vi "Autonomous.vi"   [LabVIEW 2018]
doc: "This VI starts when autonomous period begins, and will automatically be terminated when it ends. You can carry out timed or sensor driven operations directly to I/O or to subsystems without needing to return to the caller."
uses:
  <vilib>/Rock Robotics/WPI/DriverStation/WPI_DriverStationDerivedRobotMode.ctl
  <vilib>/Rock Robotics/Network Tables/NT Read String.vi
  Auton/Auton Kill Switch.vi
types:
  T1 = typedef "ADIS16470 Device Reference.ctl" = cluster{"DevStatus":errorcluster, "Hardware Config":T2, "End Calibration":refnum<notifier>, "Calibration Complete":refnum<notifier>, "Data FIFO":refnum<k33>, "Status FIFO":refnum<k33>, "Last Value Reference":refnum<data-value>, "Sychronous Process VI":T6, "Cmd FIFO":refnum<k33>}
  T2 = typedef "ADIS16470 Hardware Configuration.ctl" = cluster{"SPI Clock Rate (Hz)":dbl, "IMU SPI Mode (3)":T3, "IMU Reset Pin":T4, "IMU SPI Bus":T5, "IMU Data Ready Pin":T4}
  T3 = typedef "WPI_SPIMode.ctl" = enum16{"Mode 0 (Clk Idle Low,Sample on Leading)", "Mode 1 (Clk Idle Low,Sample on Trailing)", "Mode 2 (Clk Idle High,Sample on Leading)", "Mode 3 (Clk Idle High,Sample on Trailing)"}
  T4 = typedef "FPGA_DIOChannel.ctl" = enum8{"DIO 0", "DIO 1", "DIO 2", "DIO 3", "DIO 4", "DIO 5", "DIO 6", "DIO 7", "DIO 8", "DIO 9", "DIO MXP 0", "DIO MXP 1", "DIO MXP 2", "DIO MXP 3", "DIO MXP 4", "DIO MXP 5", "DIO MXP 6", "DIO MXP 7", "DIO MXP 8", "DIO MXP 9", "DIO MXP 10", "DIO MXP 11", "DIO MXP 12", "DIO MXP 13", "DIO MXP 14", "DIO MXP 15", "SPI Port CS1", "SPI Port CS2", "SPI Port CS3", "SPI Port MISO", "SPI Port MOSI", "Invalid"}
  T5 = typedef "spi_bus.ctl" = enum16{"SPI On-Board, CS0", "SPI On-Board, CS1", "SPI On-Board, CS2", "SPI On-Board, CS3", "SPI MXP", "Invalid"}
  T6 = typedef "ADIS16470 Process.ctl" = refnum<vi>
  T7 = typedef "ADIS16470 Status.ctl" = cluster{"Calibrated?":bool}
  T8 = typedef "WPI_DriverStationDerivedRobotMode.ctl" = enum16{"Init", "Execute", "Stop"}
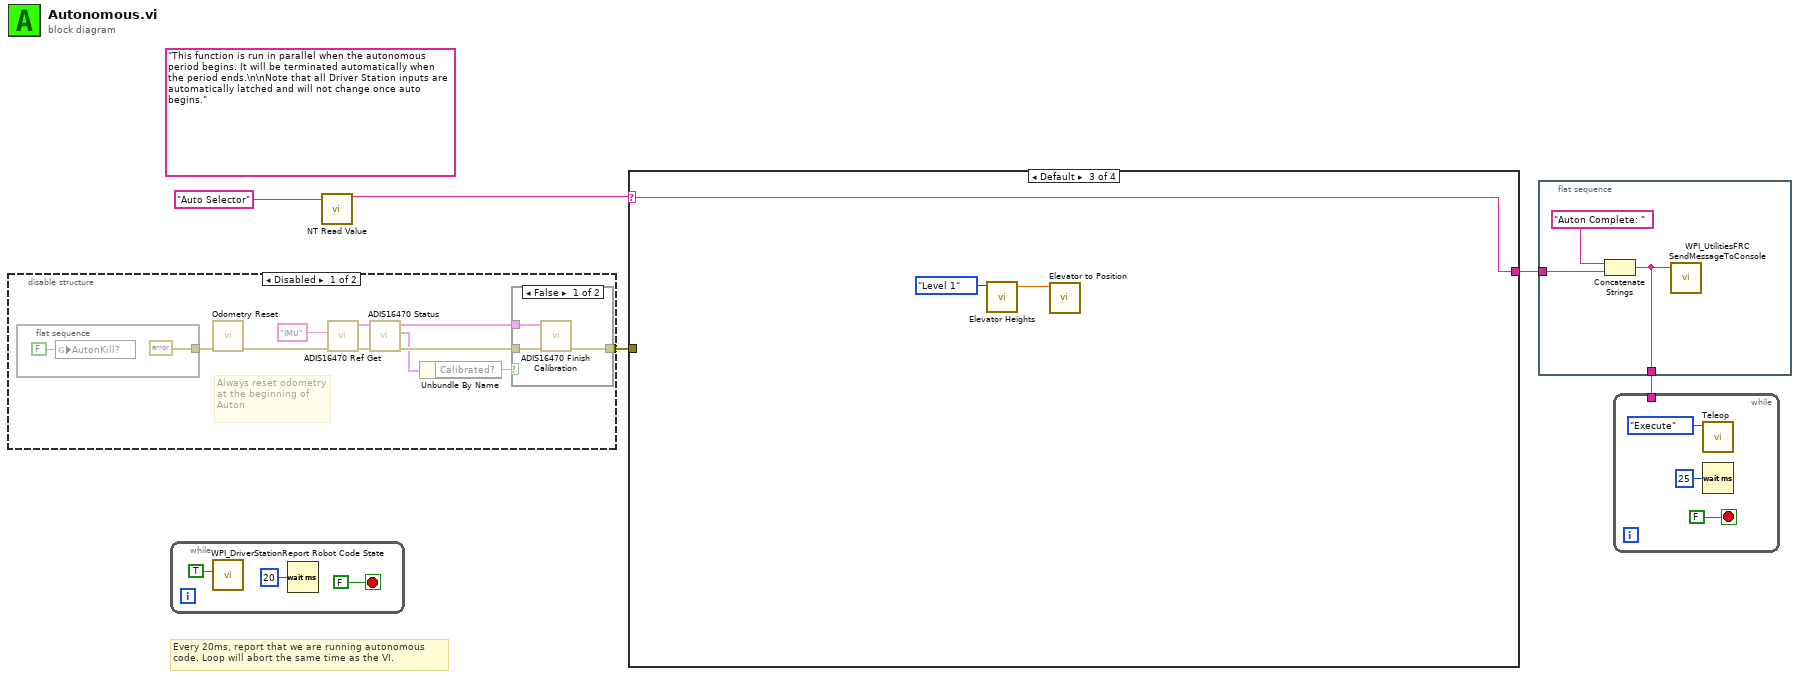
[diagram p0: block diagram]
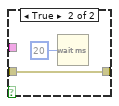
[diagram p2: hidden frame]
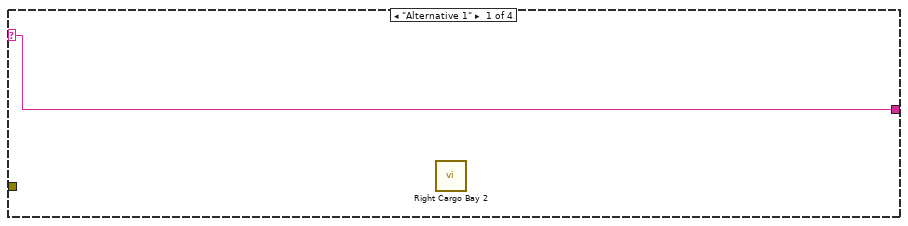
[diagram p4: hidden frame]
diagram:
  (unwired) "This function is run in parallel when the autonomous period begins. It will be terminated automatically when the period ends.\n\nNote that all Driver Station inputs are automatically latched and will not change once auto begins."
  # "Every 20ms, report that we are running autonomous\ncode. Loop will abort the same time as the VI."
  n1 = disable-structure shown="Disabled" {
    disable-tunnel: [w15 _] -> w4
    frame Disabled {
      # "Always reset odometry at the beginning of Auton"
      n2 = flat-sequence {
        tunnel: [errorcluster {"status"=FALSE, "code"=0, "source"=""} ("error in (no error)")] -> w12
        frame #0 {
          n3 = global write "Auton Kill Switch.vi" "AutonKill?"(FALSE ("AutonKill?")) -> ()
        }
      }
      n4 = call "Odometry Reset.vi"("error in (no error)"=w12) -> ("error out"=w13:errorcluster)  [unwired: 10 in]
      n5 = call "ADIS16470 Ref Get.vi"("error in (no error)"=w13, "refnum name"="IMU") -> ("error out"=w11:errorcluster, "ADIS16470 Ref"=w8:T1)  [unwired: 8 in]
      n6 = call "ADIS16470 Status.vi"("error in (no error)"=w11, "ADIS16470DevRef"=w8) -> ("error out"=w10:errorcluster, "ADIS16470 Status"=w7:T7, "ADIS16470DevRef"=w9:T1)  [unwired: 7 in]
      n7 = Unbundle By Name(w7) -> ("Calibrated?"=w6:bool)
      n8 = case shown="False" w6 {
        tunnel: [w18 w20] -> w15
        tunnel: w10 -> [w17 w20]
        tunnel: w9 -> [w16 _]
        frame False {
          n9 = call "ADIS16470 Finish Calibration.vi"("error in (no error)"=w17, "ADIS16470DevRef in"=w16) -> ("error out"=w18:errorcluster)  [unwired: 8 in, 1 out]
        }
        frame True {
          n10 = Wait (ms)(milliseconds to wait=u32 20) -> ()  [unwired: 1 out]
        }
      }
    }
    frame Enabled {
    }
  }
  n11 = while {
    stop <- FALSE stop-if-true
    n12 = call <vilib>:"WPI_DriverStationReport Robot Code State.vi"("Autonomous"=TRUE) -> ()  [unwired: 10 in, 1 out]
    n13 = Wait (ms)(milliseconds to wait=u32 20) -> ()  [unwired: 1 out]
  }
  n14 = call-poly <vilib>:"NT Read Value.vi"("Name"="Auto Selector") -> ("String"=w2:string)  [unwired: 9 in, 1 out]
  n15 = case shown="Default" w2 {
    selector: w2 -> [w26 w27 w30 w31]
    tunnel: w4 -> [_ _ _ _]
    tunnel: [w26 w27 w30 w31] -> w3
    frame "Alternative 1" {
      n16 = call "Right Cargo Bay 2.vi"() -> ()  [unwired: 12 in]
    }
    frame "Backup NT Auton" {
    }
    frame Default {
      n17 = call "Elevator Heights.vi"("Level"=enum16{"Level 1", "Level 2", "Level 3"}."Level 1") -> ("Height"=w29:dbl)  [unwired: 9 in, 1 out]
      n18 = call "Elevator to Position.vi"("Elevator Height"=w29) -> ()  [unwired: 10 in, 1 out]
    }
    frame "Alternative 2" {
    }
  }
  n19 = flat-sequence {
    tunnel: w3 -> [w33]
    tunnel: [w32] -> w1
    frame #0 {
      n20 = Concatenate Strings("Auton Complete: " ("Message"), w33) -> (w32:string)
      n21 = call <vilib>:"WPI_UtilitiesFRC SendMessageToConsole.vi"("Message"=w32) -> ()  [unwired: 14 in, 1 out]
    }
  }
  n22 = while {
    tunnel: w1 -> [_]
    stop <- FALSE stop-if-true
    n23 = call "Teleop.vi"("Call Context"=WPI_DriverStationDerivedRobotMode."Execute") -> ()  [unwired: 11 in]
    n24 = Wait (ms)(milliseconds to wait=u32 25) -> ()  [unwired: 1 out]
  }
